vi "weather_update.vi"(2 "error in":errorcluster, 3 "Weather Configuration":string="{\n  \"set_profile\": \"CloudySunset\",\n  \"profiles\": [\n    {\n      \"id\": \"Default\",\n      \"SunPolarAngle\": 44.586,\n      \"SunAzimuthAngle\": 174,\n      \"SunBrightness\": 50,\n      \"SunDirectionalLightIntensity\": 15.092,\n      \"SunDirectionalLightColor\": {\n        \"R\": 255.0,\n        \"G\": 239.0,\n        \"B\": 194.0,\n        \"A\": 1.0\n      },\n      \"SunIndirectLightIntensity\": 6,\n      \"CloudOpacity\": 16.296,\n      \"HorizontFalloff\": 3,\n      \"ZenithColor\": {\n        \"R\": 0.034046,\n        \"G\": 0.109247,\n        \"B\": 0.295,\n        \"A\": 1.0\n      },\n      \"HorizonColor\": {\n        \"R\": 0.659853, \"G\": 0.862215, \"B\": 1.0, \"A\": 1.0\n      },\n      \"CloudColor\": {\n        \"R\": 0.855778, \"G\": 0.919005, \"B\": 1.0, \"A\": 1.0\n      },\n      \"OverallSkyColor\": {\n        \"R\": 1.0, \"G\": 1.0, \"B\": 1.0, \"A\": 1.0\n      },\n      \"SkyLightIntensity\": 5.505,\n      \"SkyLightColor\": {\n        \"R\":0.149650, \"G\":0.161819, \"B\":0.205000, \"A\":0.000000\n      },\n      \"bPrecipitation\": false,\n      \"PrecipitationType\": \"Rain\",\n      \"PrecipitationAmount\": 0,\n      \"PrecipitationAccumulation\": 0,\n      \"bWind\": false,\n      \"WindIntensity\": 20,\n      \"WindAngle\": 0,\n      \"bOverrideCameraPostProcessParameters\": true,\n      \"CameraPostProcessParameters\": {\n        \"AutoExposureMethod\": \"Histogram\",\n        \"AutoExposureMinBrightness\": 0.27,\n        \"AutoExposureMaxBrightness\": 5,\n        \"AutoExposureBias\": -3.5\n      }\n    },\n    {\n      \"id\": \"ClearNoon\",\n      \"SunPolarAngle\": 44.586,\n      \"SunAzimuthAngle\": 174,\n      \"SunBrightness\": 50,\n      \"SunDirectionalLightIntensity\": 34.286,\n      \"SunDirectionalLightColor\": {\"R\":255.000000, \"G\":239.000000, \"B\":194.000000, \"A\":1.0},\n      \"SunIndirectLightIntensity\": 6,\n      \"CloudOpacity\": 16.296,\n      \"HorizontFalloff\": 3,\n      \"ZenithColor\": {\"R\":0.034046, \"G\":0.109247, \"B\":0.295000, \"A\":1.0},\n      \"HorizonColor\": {\"R\":0.659853, \"G\":0.862215, \"B\":1.0, \"A\":1.0},\n      \"CloudColor\": {\"R\":0.855778, \"G\":0.919005, \"B\":1.0, \"A\":1.0},\n      \"OverallSkyColor\": {\"R\":1.0, \"G\":1.0, \"B\":1.0, \"A\":1.0},\n      \"SkyLightIntensity\": 10,\n      \"SkyLightColor\": {\"R\":0.195000, \"G\":0.193979, \"B\":0.152151, \"A\":0.000000},\n      \"bPrecipitation\": false,\n      \"PrecipitationType\": \"Rain\",\n      \"PrecipitationAmount\": 0,\n      \"PrecipitationAccumulation\": 0,\n      \"bWind\": false,\n      \"WindIntensity\": 20,\n      \"WindAngle\": 0,\n      \"bOverrideCameraPostProcessParameters\": true,\n      \"CameraPostProcessParameters\":{\n        \"AutoExposureMethod\": \"Histogram\",\n        \"AutoExposureMinBrightness\": 0.27,\n        \"AutoExposureMaxBrightness\": 5,\n        \"AutoExposureBias\": -3.5\n      }\n    },\n    {\n      \"id\": \"CloudyNoon\",\n      \"SunPolarAngle\": 44.586,\n      \"SunAzimuthAngle\": 174,\n      \"SunBrightness\": 0,\n      \"SunDirectionalLightIntensity\": 1.835,\n      \"SunDirectionalLightColor\": {\"R\":1.0, \"G\":0.862295, \"B\":0.475000, \"A\":1.0},\n      \"SunIndirectLightIntensity\": 6,\n      \"CloudOpacity\": 18.431,\n      \"HorizontFalloff\": 3,\n      \"ZenithColor\": {\"R\":1.0, \"G\":1.0, \"B\":1.0, \"A\":1.0},\n      \"HorizonColor\": {\"R\":0.169000, \"G\":0.187443, \"B\":0.200000, \"A\":1.0},\n      \"CloudColor\": {\"R\":0.143627, \"G\":0.159235, \"B\":0.190000, \"A\":1.0},\n      \"OverallSkyColor\": {\"R\":1.0, \"G\":1.0, \"B\":1.0, \"A\":1.0},\n      \"SkyLightIntensity\": 16.514,\n      \"SkyLightColor\": {\"R\":0.100887, \"G\":0.106803, \"B\":0.145000, \"A\":0.000000},\n      \"bPrecipitation\": false,\n      \"PrecipitationType\": \"Rain\",\n      \"PrecipitationAmount\": 0,\n      \"PrecipitationAccumulation\": 0,\n      \"bWind\": false,\n      \"WindIntensity\": 20,\n      \"WindAngle\": 0,\n      \"bOverrideCameraPostProcessParameters\": true,\n      \"CameraPostProcessParameters\": {\n        \"AutoExposureMethod\": \"Histogram\",\n        \"AutoExposureMinBrightness\": 0.27,\n        \"AutoExposureMaxBrightness\": 5,\n        \"AutoExposureBias\": -3.5\n      }\n    },\n    {\n      \"id\": \"WetNoon\",\n      \"SunPolarAngle\": 44.586,\n      \"SunAzimuthAngle\": 174,\n      \"SunBrightness\": 3.67,\n      \"SunDirectionalLightIntensity\": 20.184,\n      \"SunDirectionalLightColor\": {\"R\":1.0, \"G\":0.862295, \"B\":0.475000, \"A\":1.0},\n      \"SunIndirectLightIntensity\": 6,\n      \"CloudOpacity\": 17.431,\n      \"HorizontFalloff\": 5.752,\n      \"ZenithColor\": {\"R\":0.000000, \"G\":0.085618, \"B\":0.715000, \"A\":1.0},\n      \"HorizonColor\": {\"R\":0.532350, \"G\":0.590445, \"B\":0.630000, \"A\":1.0},\n      \"CloudColor\": {\"R\":0.143627, \"G\":0.159235, \"B\":0.190000, \"A\":1.0},\n      \"OverallSkyColor\": {\"R\":0.660000, \"G\":0.630413, \"B\":0.518100, \"A\":1.0},\n      \"SkyLightIntensity\": 14.679,\n      \"SkyLightColor\": {\"R\":0.135000, \"G\":0.120150, \"B\":0.075600, \"A\":0.000000},\n      \"bPrecipitation\": true,\n      \"PrecipitationType\": \"Rain\",\n      \"PrecipitationAmount\": 0,\n      \"PrecipitationAccumulation\": 54.128,\n      \"bWind\": false,\n      \"WindIntensity\": 20,\n      \"WindAngle\": 0,\n      \"bOverrideCameraPostProcessParameters\": true,\n      \"CameraPostProcessParameters\": {\n        \"AutoExposureMethod\": \"Histogram\",\n        \"AutoExposureMinBrightness\": 0.27,\n        \"AutoExposureMaxBrightness\": 5,\n        \"AutoExposureBias\": -3.5\n      }\n    },\n    {\n      \"id\": \"WetCloudyNoon\",\n      \"SunPolarAngle\": 44.586,\n      \"SunAzimuthAngle\": 174,\n      \"SunBrightness\": 0,\n      \"SunDirectionalLightIntensity\": 1.835,\n      \"SunDirectionalLightColor\": {\"R\":1.0, \"G\":0.862295, \"B\":0.475000, \"A\":1.0},\n      \"SunIndirectLightIntensity\": 6,\n      \"CloudOpacity\": 18.431,\n      \"HorizontFalloff\": 3,\n      \"ZenithColor\": {\"R\":1.0, \"G\":1.0, \"B\":1.0, \"A\":1.0},\n      \"HorizonColor\": {\"R\":0.000000, \"G\":0.000000, \"B\":0.000000, \"A\":1.0},\n      \"CloudColor\": {\"R\":0.230559, \"G\":0.255614, \"B\":0.305000, \"A\":1.0},\n      \"OverallSkyColor\": {\"R\":0.660000, \"G\":0.630413, \"B\":0.518100, \"A\":1.0},\n      \"SkyLightIntensity\": 25.688,\n      \"SkyLightColor\": {\"R\":0.135000, \"G\":0.120150, \"B\":0.075600, \"A\":0.000000},\n      \"bPrecipitation\": true,\n      \"PrecipitationType\": \"Rain\",\n      \"PrecipitationAmount\": 0,\n      \"PrecipitationAccumulation\": 47.706,\n      \"bWind\": false,\n      \"WindIntensity\": 20,\n      \"WindAngle\": 0,\n      \"bOverrideCameraPostProcessParameters\": true,\n      \"CameraPostProcessParameters\": {\n        \"AutoExposureMethod\": \"Histogram\",\n        \"AutoExposureMinBrightness\": 0.27,\n        \"AutoExposureMaxBrightness\": 5,\n        \"AutoExposureBias\": -3.5\n      }\n    },\n    {\n      \"id\": \"MidRainyNoon\",\n      \"SunPolarAngle\": 44.586,\n      \"SunAzimuthAngle\": 174,\n      \"SunBrightness\": 0,\n      \"SunDirectionalLightIntensity\": 1.33,\n      \"SunDirectionalLightColor\": {\"R\":255.000000, \"G\":239.000000, \"B\":194.000000, \"A\":1.0},\n      \"SunIndirectLightIntensity\": 6,\n      \"CloudOpacity\": 18.431,\n      \"HorizontFalloff\": 3,\n      \"ZenithColor\": {\"R\":0.370000, \"G\":0.370000, \"B\":0.370000, \"A\":1.0},\n      \"HorizonColor\": {\"R\":0.169000, \"G\":0.187443, \"B\":0.200000, \"A\":1.0},\n      \"CloudColor\": {\"R\":0.042789, \"G\":0.045950, \"B\":0.050000, \"A\":1.0},\n      \"OverallSkyColor\": {\"R\":1.0, \"G\":1.0, \"B\":1.0, \"A\":1.0},\n      \"SkyLightIntensity\": 21.147,\n      \"SkyLightColor\": {\"R\":0.119882, \"G\":0.121557, \"B\":0.170000, \"A\":0.000000},\n      \"bPrecipitation\": true,\n      \"PrecipitationType\": \"Rain\",\n      \"PrecipitationAmount\": 40,\n      \"PrecipitationAccumulation\": 50,\n      \"bWind\": false,\n      \"WindIntensity\": 40,\n      \"WindAngle\": 0,\n      \"bOverrideCameraPostProcessParameters\": true,\n      \"CameraPostProcessParameters\": {\n        \"AutoExposureMethod\": \"Histogram\",\n        \"AutoExposureMinBrightness\": 0.27,\n        \"AutoExposureMaxBrightness\": 5,\n        \"AutoExposureBias\": -3.5\n      }\n    },\n    {\n      \"id\": \"HardRainNoon\",\n      \"SunPolarAngle\": 44.586,\n      \"SunAzimuthAngle\": 174,\n      \"SunBrightness\": 0,\n      \"SunDirectionalLightIntensity\": 1.33,\n      \"SunDirectionalLightColor\": {\"R\":255.000000, \"G\":239.000000, \"B\":194.000000, \"A\":1.0},\n      \"SunIndirectLightIntensity\": 6,\n      \"CloudOpacity\": 18.431,\n      \"HorizontFalloff\": 3,\n      \"ZenithColor\": {\"R\":0.580000, \"G\":0.580000, \"B\":0.580000, \"A\":1.0},\n      \"HorizonColor\": {\"R\":0.169000, \"G\":0.187443, \"B\":0.200000, \"A\":1.0},\n      \"CloudColor\": {\"R\":0.089857, \"G\":0.096495, \"B\":0.105000, \"A\":1.0},\n      \"OverallSkyColor\": {\"R\":1.0, \"G\":1.0, \"B\":1.0, \"A\":1.0},\n      \"SkyLightIntensity\": 37.66,\n      \"SkyLightColor\": {\"R\":0.126934, \"G\":0.128707, \"B\":0.180000, \"A\":0.000000},\n      \"bPrecipitation\": true,\n      \"PrecipitationType\": \"Rain\",\n      \"PrecipitationAmount\": 80,\n      \"PrecipitationAccumulation\": 87.248,\n      \"bWind\": false,\n      \"WindIntensity\": 40,\n      \"WindAngle\": 0,\n      \"bOverrideCameraPostProcessParameters\": true,\n      \"CameraPostProcessParameters\": {\n        \"AutoExposureMethod\": \"Histogram\",\n        \"AutoExposureMinBrightness\": 0.27,\n        \"AutoExposureMaxBrightness\": 5,\n        \"AutoExposureBias\": -3.5\n      }\n    },\n    {\n      \"id\":\"SoftRainNoon\",\n      \"SunPolarAngle\": 44.586,\n      \"SunAzimuthAngle\": 174,\n      \"SunBrightness\": 0,\n      \"SunDirectionalLightIntensity\": 1.33,\n      \"SunDirectionalLightColor\": {\"R\":255.000000, \"G\":239.000000, \"B\":194.000000, \"A\":1.0},\n      \"SunIndirectLightIntensity\": 6,\n      \"CloudOpacity\": 18.431,\n      \"HorizontFalloff\": 3,\n      \"ZenithColor\": {\"R\":1.0, \"G\":1.0, \"B\":1.0, \"A\":1.0},\n      \"HorizonColor\": {\"R\":0.169000, \"G\":0.187443, \"B\":0.200000, \"A\":1.0},\n      \"CloudColor\": {\"R\":0.440725, \"G\":0.473285, \"B\":0.515000, \"A\":1.0},\n      \"OverallSkyColor\": {\"R\":1.0, \"G\":1.0, \"B\":1.0, \"A\":1.0},\n      \"SkyLightIntensity\": 3,\n      \"SkyLightColor\": {\"R\":0.525365, \"G\":0.532706, \"B\":0.745000, \"A\":0.000000},\n      \"bPrecipitation\": true,\n      \"PrecipitationType\": \"Rain\",\n      \"PrecipitationAmount\": 10.55,\n      \"PrecipitationAccumulation\": 61.927,\n      \"bWind\": false,\n      \"WindIntensity\": 20,\n      \"WindAngle\": 0,\n      \"bOverrideCameraPostProcessParameters\": true,\n      \"CameraPostProcessParameters\": {\n        \"AutoExposureMethod\": \"Histogram\",\n        \"AutoExposureMinBrightness\": 0.27,\n        \"AutoExposureMaxBrightness\": 5,\n        \"AutoExposureBias\": -3.5\n      }\n    },\n    {\n      \"id\": \"ClearSunset\",\n      \"SunPolarAngle\": 86,\n      \"SunAzimuthAngle\": 174,\n      \"SunBrightness\": 1.835,\n      \"SunDirectionalLightIntensity\": 50,\n      \"SunDirectionalLightColor\": {\"R\":0.810000, \"G\":0.347470, \"B\":0.170100, \"A\":1.0},\n      \"SunIndirectLightIntensity\": 73.394,\n      \"CloudOpacity\": 27.63,\n      \"HorizontFalloff\": 0.917,\n      \"ZenithColor\": {\"R\":0.046375, \"G\":0.044100, \"B\":0.105000, \"A\":1.0},\n      \"HorizonColor\": {\"R\":0.745000, \"G\":0.219006, \"B\":0.046649, \"A\":1.0},\n      \"CloudColor\": {\"R\":1.0, \"G\":0.561587, \"B\":0.189305, \"A\":1.0},\n      \"OverallSkyColor\": {\"R\":1.0, \"G\":1.0, \"B\":1.0, \"A\":1.0},\n      \"SkyLightIntensity\": 14,\n      \"SkyLightColor\": {\"R\":0.076220, \"G\":0.074724, \"B\":0.109375, \"A\":0.000000},\n      \"bPrecipitation\": false,\n      \"PrecipitationType\": \"Rain\",\n      \"PrecipitationAmount\": 0,\n      \"PrecipitationAccumulation\": 0,\n      \"bWind\": false,\n      \"WindIntensity\": 20,\n      \"WindAngle\": 0,\n      \"bOverrideCameraPostProcessParameters\": true,\n      \"CameraPostProcessParameters\": {\n        \"AutoExposureMethod\": \"Histogram\",\n        \"AutoExposureMinBrightness\": 0.27,\n        \"AutoExposureMaxBrightness\": 5,\n        \"AutoExposureBias\": -3.5\n      }\n    },\n    {\n      \"id\": \"CloudySunset\",\n      \"SunPolarAngle\": 86,\n      \"SunAzimuthAngle\": 174,\n      \"SunBrightness\": 67.89,\n      \"SunDirectionalLightIntensity\": 6.422,\n      \"SunDirectionalLightColor\": {\"R\":0.810000, \"G\":0.347162, \"B\":0.083003, \"A\":1.0},\n      \"SunIndirectLightIntensity\": 6,\n      \"CloudOpacity\": 28.869,\n      \"HorizontFalloff\": 1.165,\n      \"ZenithColor\": {\"R\":0.046375, \"G\":0.044100, \"B\":0.105000, \"A\":1.0},\n      \"HorizonColor\": {\"R\":1.0, \"G\":0.007579, \"B\":0.000000, \"A\":1.0},\n      \"CloudColor\": {\"R\":1.0, \"G\":0.518982, \"B\":0.175000, \"A\":1.0},\n      \"OverallSkyColor\": {\"R\":0.410000, \"G\":0.410000, \"B\":0.410000, \"A\":1.0},\n      \"SkyLightIntensity\": 36.239,\n      \"SkyLightColor\": {\"R\":0.193050, \"G\":0.195113, \"B\":0.270000, \"A\":0.000000},\n      \"bPrecipitation\": false,\n      \"PrecipitationType\": \"Rain\",\n      \"PrecipitationAmount\": 0,\n      \"PrecipitationAccumulation\": 0,\n      \"bWind\": false,\n      \"WindIntensity\": 20,\n      \"WindAngle\": 0,\n      \"bOverrideCameraPostProcessParameters\": true,\n      \"CameraPostProcessParameters\": {\n        \"AutoExposureMethod\": \"Histogram\",\n        \"AutoExposureMinBrightness\": 0.27,\n        \"AutoExposureMaxBrightness\": 5,\n        \"AutoExposureBias\": -3.5\n      }\n    },\n    {\n      \"id\": \"WetSunset\",\n      \"SunPolarAngle\": 86,\n      \"SunAzimuthAngle\": 174,\n      \"SunBrightness\": 0,\n      \"SunDirectionalLightIntensity\": 25.688,\n      \"SunDirectionalLightColor\": {\"R\":0.810000, \"G\":0.347162, \"B\":0.083003, \"A\":1.0},\n      \"SunIndirectLightIntensity\": 6,\n      \"CloudOpacity\": 17.596,\n      \"HorizontFalloff\": 1.165,\n      \"ZenithColor\": {\"R\":0.046375, \"G\":0.044100, \"B\":0.105000, \"A\":1.0},\n      \"HorizonColor\": {\"R\":0.695000, \"G\":0.379445, \"B\":0.150922, \"A\":1.0},\n      \"CloudColor\": {\"R\":1.0, \"G\":0.561587, \"B\":0.189305, \"A\":1.0},\n      \"OverallSkyColor\": {\"R\":1.0, \"G\":1.0, \"B\":1.0, \"A\":1.0},\n      \"SkyLightIntensity\": 66.972,\n      \"SkyLightColor\": {\"R\":0.113887, \"G\":0.110000, \"B\":0.200000, \"A\":0.000000},\n      \"bPrecipitation\": true,\n      \"PrecipitationType\": \"Rain\",\n      \"PrecipitationAmount\": 0,\n      \"PrecipitationAccumulation\": 65.046,\n      \"bWind\": false,\n      \"WindIntensity\": 20,\n      \"WindAngle\": 0,\n      \"bOverrideCameraPostProcessParameters\": true,\n      \"CameraPostProcessParameters\": {\n        \"AutoExposureMethod\": \"Histogram\",\n        \"AutoExposureMinBrightness\": 0.27,\n        \"AutoExposureMaxBrightness\": 5,\n        \"AutoExposureBias\": -3.5\n      }\n    },\n    {\n      \"id\": \"WetCloudySunset\",\n      \"SunPolarAngle\": 86,\n      \"SunAzimuthAngle\": 174,\n      \"SunBrightness\": 67.89,\n      \"SunDirectionalLightIntensity\": 25.688,\n      \"SunDirectionalLightColor\": {\"R\":0.810000, \"G\":0.347162, \"B\":0.083003, \"A\":1.0},\n      \"SunIndirectLightIntensity\": 6,\n      \"CloudOpacity\": 15,\n      \"HorizontFalloff\": 1.165,\n      \"ZenithColor\": {\"R\":0.046375, \"G\":0.044100, \"B\":0.105000, \"A\":1.0},\n      \"HorizonColor\": {\"R\":0.695000, \"G\":0.379445, \"B\":0.150922, \"A\":1.0},\n      \"CloudColor\": {\"R\":1.0, \"G\":0.561587, \"B\":0.189305, \"A\":1.0},\n      \"OverallSkyColor\": {\"R\":1.0, \"G\":1.0, \"B\":1.0, \"A\":1.0},\n      \"SkyLightIntensity\": 50,\n      \"SkyLightColor\": {\"R\":0.083625, \"G\":0.081983, \"B\":0.120000, \"A\":0.000000},\n      \"bPrecipitation\": false,\n      \"PrecipitationType\": \"Rain\",\n      \"PrecipitationAmount\": 0,\n      \"PrecipitationAccumulation\": 0,\n      \"bWind\": false,\n      \"WindIntensity\": 20,\n      \"WindAngle\": 0,\n      \"bOverrideCameraPostProcessParameters\": true,\n      \"CameraPostProcessParameters\": {\n        \"AutoExposureMethod\": \"Histogram\",\n        \"AutoExposureMinBrightness\": 0.27,\n        \"AutoExposureMaxBrightness\": 5,\n        \"AutoExposureBias\": -3.5\n      }\n    },\n    {\n      \"id\": \"MidRainSunset\",\n      \"SunPolarAngle\": 86,\n      \"SunAzimuthAngle\": 174,\n      \"SunBrightness\": 12.381,\n      \"SunDirectionalLightIntensity\": 5.714,\n      \"SunDirectionalLightColor\": {\"R\":0.810000, \"G\":0.347162, \"B\":0.083003, \"A\":1.0},\n      \"SunIndirectLightIntensity\": 6,\n      \"CloudOpacity\": 17.143,\n      \"HorizontFalloff\": 1.835,\n      \"ZenithColor\": {\"R\":0.317708, \"G\":0.208096, \"B\":0.260868, \"A\":1.0},\n      \"HorizonColor\": {\"R\":1.0, \"G\":0.590000, \"B\":0.000000, \"A\":1.0},\n      \"CloudColor\": {\"R\":0.555000, \"G\":0.290880, \"B\":0.066600, \"A\":1.0},\n      \"OverallSkyColor\": {\"R\":1.0, \"G\":1.0, \"B\":1.0, \"A\":1.0},\n      \"SkyLightIntensity\": 6.667,\n      \"SkyLightColor\": {\"R\":0.214844, \"G\":0.273773, \"B\":0.750000, \"A\":0.000000},\n      \"bPrecipitation\": true,\n      \"PrecipitationType\": \"Rain\",\n      \"PrecipitationAmount\": 37.156,\n      \"PrecipitationAccumulation\": 88.073,\n      \"bWind\": false,\n      \"WindIntensity\": 20,\n      \"WindAngle\": 0,\n      \"bOverrideCameraPostProcessParameters\": true,\n      \"CameraPostProcessParameters\": {\n        \"AutoExposureMethod\": \"Histogram\",\n        \"AutoExposureMinBrightness\": 0.27,\n        \"AutoExposureMaxBrightness\": 5,\n        \"AutoExposureBias\": -3.5\n      }\n    },\n    {\n      \"id\": \"HardRainSunset\",\n      \"SunPolarAngle\": 86,\n      \"SunAzimuthAngle\": 174,\n      \"SunBrightness\": 0.952,\n      \"SunDirectionalLightIntensity\": 3.063,\n      \"SunDirectionalLightColor\": {\"R\":0.810000, \"G\":0.347162, \"B\":0.083003, \"A\":1.0},\n      \"SunIndirectLightIntensity\": 6,\n      \"CloudOpacity\": 17.37,\n      \"HorizontFalloff\": 1.835,\n      \"ZenithColor\": {\"R\":0.307292, \"G\":0.161669, \"B\":0.123237, \"A\":1.0},\n      \"HorizonColor\": {\"R\":0.453125, \"G\":0.297809, \"B\":0.228923, \"A\":1.0},\n      \"CloudColor\": {\"R\":0.416667, \"G\":0.288257, \"B\":0.189558, \"A\":1.0},\n      \"OverallSkyColor\": {\"R\":1.0, \"G\":0.736403, \"B\":0.487039, \"A\":1.0},\n      \"SkyLightIntensity\": 5.81,\n      \"SkyLightColor\": {\"R\":0.500000, \"G\":0.383356, \"B\":0.250000, \"A\":0.000000},\n      \"bPrecipitation\": true,\n      \"PrecipitationType\": \"Rain\",\n      \"PrecipitationAmount\": 84.862,\n      \"PrecipitationAccumulation\": 100,\n      \"bWind\": false,\n      \"WindIntensity\": 20,\n      \"WindAngle\": 0,\n      \"bOverrideCameraPostProcessParameters\": true,\n      \"CameraPostProcessParameters\": {\n        \"AutoExposureMethod\": \"Histogram\",\n        \"AutoExposureMinBrightness\": 0.27,\n        \"AutoExposureMaxBrightness\": 5,\n        \"AutoExposureBias\": -3.5\n      }\n    },\n    {\n      \"id\": \"SoftRainSunset\",\n      \"SunPolarAngle\": 86,\n      \"SunAzimuthAngle\": 174,\n      \"SunBrightness\": 13.761,\n      \"SunDirectionalLightIntensity\": 12.587,\n      \"SunDirectionalLightColor\": {\"R\":0.810000, \"G\":0.347162, \"B\":0.083003, \"A\":1.0},\n      \"SunIndirectLightIntensity\": 6,\n      \"CloudOpacity\": 34.513,\n      \"HorizontFalloff\": 1.835,\n      \"ZenithColor\": {\"R\":0.360000, \"G\":0.125625, \"B\":0.142175, \"A\":1.0},\n      \"HorizonColor\": {\"R\":1.0, \"G\":0.590000, \"B\":0.000000, \"A\":1.0},\n      \"CloudColor\": {\"R\":0.296875, \"G\":0.169776, \"B\":0.061849, \"A\":1.0},\n      \"OverallSkyColor\": {\"R\":1.0, \"G\":1.0, \"B\":1.0, \"A\":1.0},\n      \"SkyLightIntensity\": 7.339,\n      \"SkyLightColor\": {\"R\":0.458070, \"G\":0.394209, \"B\":0.750000, \"A\":0.000000},\n      \"bPrecipitation\": true,\n      \"PrecipitationType\": \"Rain\",\n      \"PrecipitationAmount\": 8.716,\n      \"PrecipitationAccumulation\": 53.211,\n      \"bWind\": false,\n      \"WindIntensity\": 20,\n      \"WindAngle\": 0,\n      \"bOverrideCameraPostProcessParameters\": true,\n      \"CameraPostProcessParameters\": {\n        \"AutoExposureMethod\": \"Histogram\",\n        \"AutoExposureMinBrightness\": 0.27,\n        \"AutoExposureMaxBrightness\": 5,\n        \"AutoExposureBias\": -3.5\n      }\n    }\n  ]\n}\n", 4 "simx in":T1={"Config"={"Trajectory"={"Number of frames"=0, "Frame number"=0, "Trajectory"=""}, "Weather"={"id"=""}}, "Connections"={"Simulator Connection"=refnum, "server_ip"="127.0.0.1", "Port"=0, "Sensor connections"=[]}, "Map"={"lanes"={"x"=[], "y"=[], "z"=[]}, "StartPosition"={"start_points"={"locations"=[], "rotations"=[], "type"=[]}, "StartRotation"=[], "StartLocation"=[]}, "Draw Map Size"={"Width"=0, "Height"=0}, "DrawArea"={"min_Y"=0.0, "min_X"=0.0, "Scale X"=0.0, "Scale Y"=0.0}, "Map"=bytes[0], "Map Geojson"=""}}) -> (0 "error out":errorcluster, 1 "simx out":T1={"Config"={"Trajectory"={"Number of frames"=0, "Frame number"=0, "Trajectory"=""}, "Weather"={"id"=""}}, "Connections"={"Simulator Connection"=refnum, "server_ip"="127.0.0.1", "Port"=0, "Sensor connections"=[]}, "Map"={"lanes"={"x"=[], "y"=[], "z"=[]}, "StartPosition"={"start_points"={"locations"=[], "rotations"=[], "type"=[]}, "StartRotation"=[], "StartLocation"=[]}, "Draw Map Size"={"Width"=0, "Height"=0}, "DrawArea"={"min_Y"=0.0, "min_X"=0.0, "Scale X"=0.0, "Scale Y"=0.0}, "Map"=bytes[0], "Map Geojson"=""}})   [LabVIEW 2019, in "Lib_Simx.lvlib"]
doc: "Sends weather configuration to the simulator."
uses:
  Lib_Simx.lvlib
  controls/simx_connection.ctl
  controls/config.ctl
  controls/trajectory.ctl
  controls/weather.ctl
  controls/connections.ctl
  controls/start_points.ctl
  <vilib>/Utility/miscctls.llb/LVBoundsTypeDef.ctl
panel:
  out "JSON string":string
  out "weather updated":bool
  out "config response":string
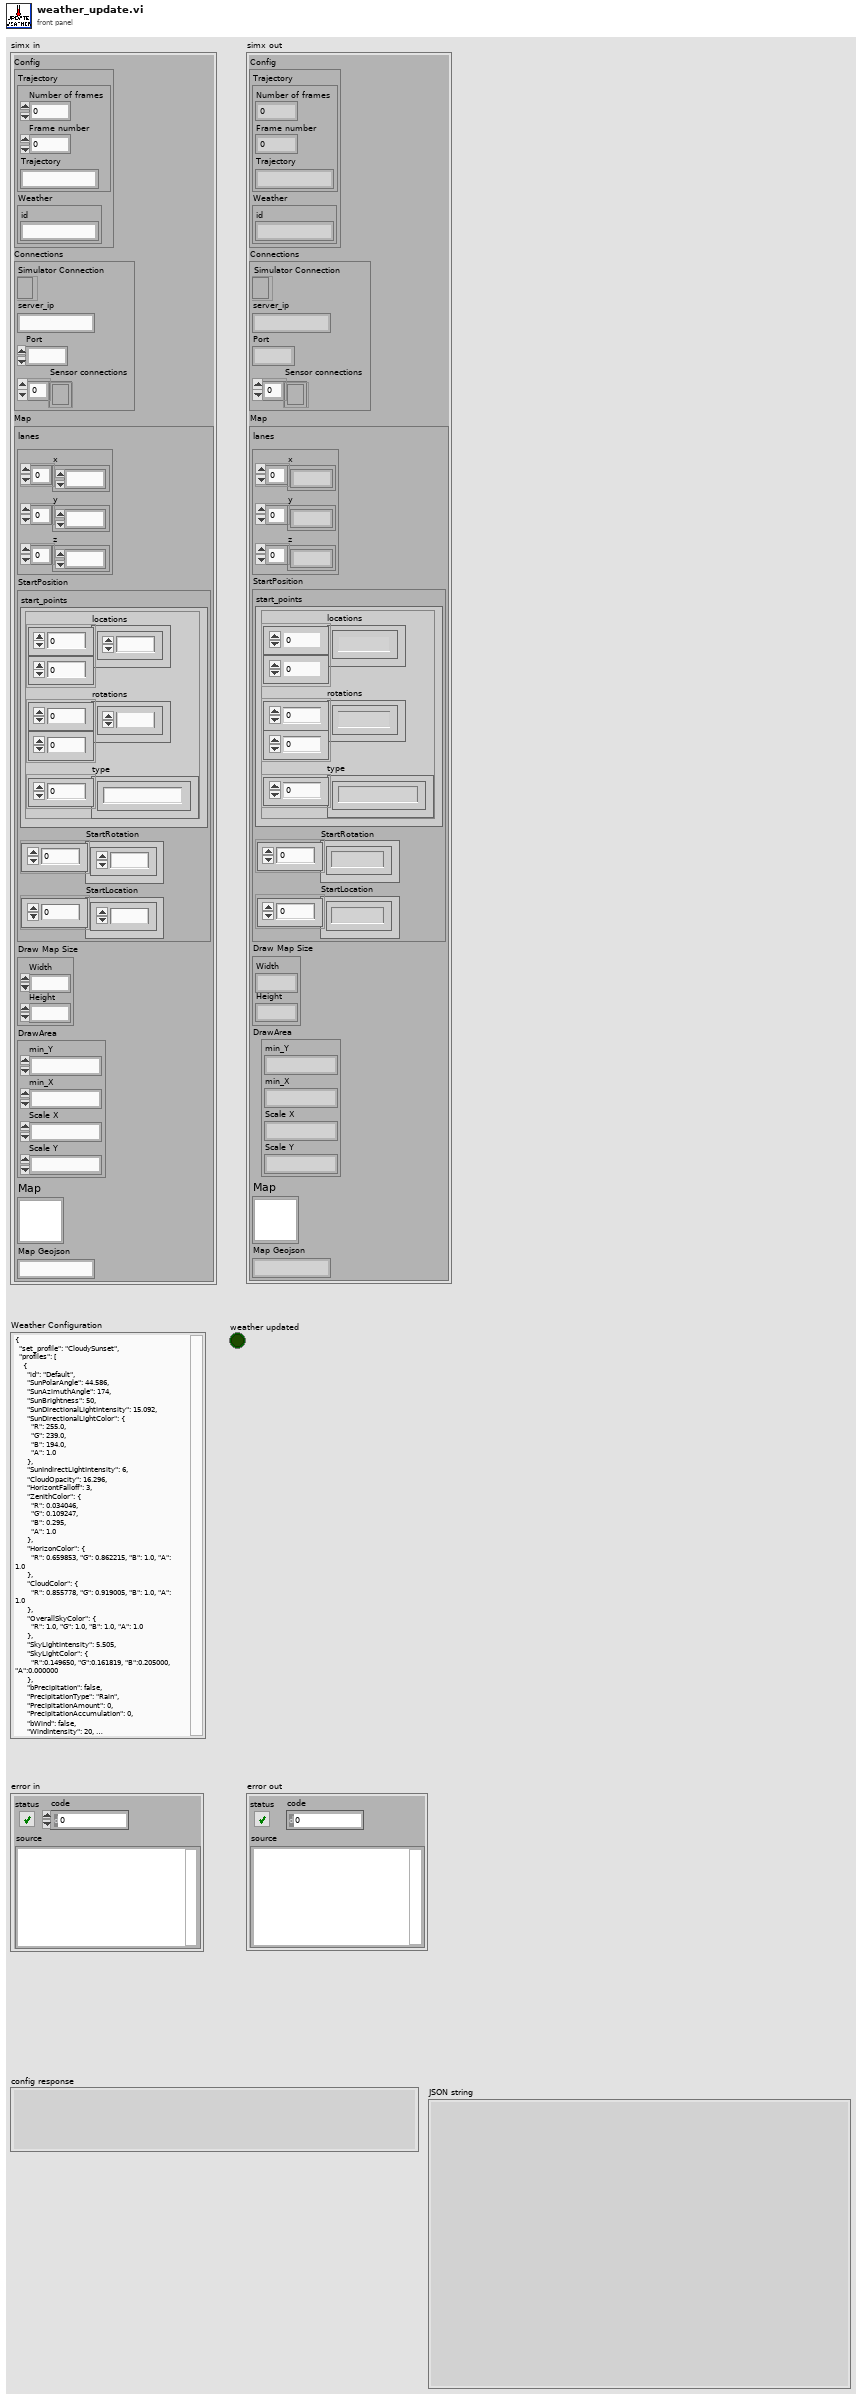
[diagram p1: front panel]
types:
  T1 = typedef "Lib_Simx.lvlib/simx_connection.ctl" = cluster{"Config":T2, "Connections":T5, "Map":cluster{"lanes":cluster{"x":dbl[], "y":dbl[], "z":dbl[]}, "StartPosition":cluster{"start_points":T6, "StartRotation":dbl[], "StartLocation":dbl[]}, "Draw Map Size":T7, "DrawArea":cluster{"min_Y":dbl, "min_X":dbl, "Scale X":dbl, "Scale Y":dbl}, "Map":picture, "Map Geojson":string}}
  T2 = typedef "Lib_Simx.lvlib/config.ctl" = cluster{"Trajectory":T3, "Weather":T4}
  T3 = typedef "Lib_Simx.lvlib/trajectory.ctl" = cluster{"Number of frames":i32, "Frame number":i32, "Trajectory":string}
  T4 = typedef "Lib_Simx.lvlib/weather.ctl" = cluster{"id":string}
  T5 = typedef "Lib_Simx.lvlib/connections.ctl" = cluster{"Simulator Connection":refnum<k5>, "server_ip":string, "Port":i32, "Sensor connections":refnum<k5>[]}
  T6 = typedef "Lib_Simx.lvlib/start_points.ctl" = cluster{"locations":dbl[][], "rotations":dbl[][], "type":string[]}
  T7 = typedef "LVBoundsTypeDef.ctl" = cluster{"Width":u32, "Height":u32}
  T8 = cluster{"set_description":string, "descriptions":cluster{"id":string, "CloudColor":cluster{"A":sgl, "B":sgl, "G":sgl, "R":sgl}, "CloudOpacity":sgl, "Day":sgl, "FogCutoffDistance":sgl, "FogDensity":sgl, "FogHeightFalloff":sgl, "FogInscatteringColor":cluster{"A":sgl, "B":sgl, "G":sgl, "R":sgl}, "FogMaxOpacity":sgl, "FogStartDistance":sgl, "HorizonColor":cluster{"A":sgl, "B":sgl, "G":sgl, "R":sgl}, "HorizonFalloff":sgl, "Hours":sgl, "IsDaylightSavingTime":bool, "Latitude":sgl, "Longitude":sgl, "Minutes":sgl, "Month":sgl, "NorthOffset":sgl, "OverallSkyColor":cluster{"A":sgl, "B":sgl, "G":sgl, "R":sgl}, "OverideTimeBasedSunAngle":bool, "PrecipitationAccumulation":sgl, "PrecipitationAmount":sgl, "PrecipitationType":string, "SecondFogDensity":sgl, "SecondFogHeightFalloff":sgl, "SecondFogHeightOffset":sgl, "Seconds":sgl, "SkyLightColor":cluster{"A":sgl, "B":sgl, "G":sgl, "R":sgl}, "SkyLightIntensity":sgl, "StarBrightness":sgl, "SunAzimuthAngle":sgl, "SunBrightness":sgl, "SunDirectionalLightColor":cluster{"A":sgl, "B":sgl, "G":sgl, "R":sgl}, "SunDirectionalLightIntensity":sgl, "SunPolarAngle":sgl, "TimeZone":sgl, "WindAngle":sgl, "WindIntensity":sgl, "Year":sgl, "ZenithColor":cluster{"A":sgl, "B":sgl, "G":sgl, "R":sgl}, "bPrecipitation":bool, "bWind":bool}[]}
  T9 = cluster{"type":string, "success":bool, "reference":i32}
  T10 = cluster{"id":string, "CloudColor":cluster{"A":sgl, "B":sgl, "G":sgl, "R":sgl}, "CloudOpacity":sgl, "Day":sgl, "FogCutoffDistance":sgl, "FogDensity":sgl, "FogHeightFalloff":sgl, "FogInscatteringColor":cluster{"A":sgl, "B":sgl, "G":sgl, "R":sgl}, "FogMaxOpacity":sgl, "FogStartDistance":sgl, "HorizonColor":cluster{"A":sgl, "B":sgl, "G":sgl, "R":sgl}, "HorizonFalloff":sgl, "Hours":sgl, "IsDaylightSavingTime":bool, "Latitude":sgl, "Longitude":sgl, "Minutes":sgl, "Month":sgl, "NorthOffset":sgl, "OverallSkyColor":cluster{"A":sgl, "B":sgl, "G":sgl, "R":sgl}, "OverideTimeBasedSunAngle":bool, "PrecipitationAccumulation":sgl, "PrecipitationAmount":sgl, "PrecipitationType":string, "SecondFogDensity":sgl, "SecondFogHeightFalloff":sgl, "SecondFogHeightOffset":sgl, "Seconds":sgl, "SkyLightColor":cluster{"A":sgl, "B":sgl, "G":sgl, "R":sgl}, "SkyLightIntensity":sgl, "StarBrightness":sgl, "SunAzimuthAngle":sgl, "SunBrightness":sgl, "SunDirectionalLightColor":cluster{"A":sgl, "B":sgl, "G":sgl, "R":sgl}, "SunDirectionalLightIntensity":sgl, "SunPolarAngle":sgl, "TimeZone":sgl, "WindAngle":sgl, "WindIntensity":sgl, "Year":sgl, "ZenithColor":cluster{"A":sgl, "B":sgl, "G":sgl, "R":sgl}, "bPrecipitation":bool, "bWind":bool}[]
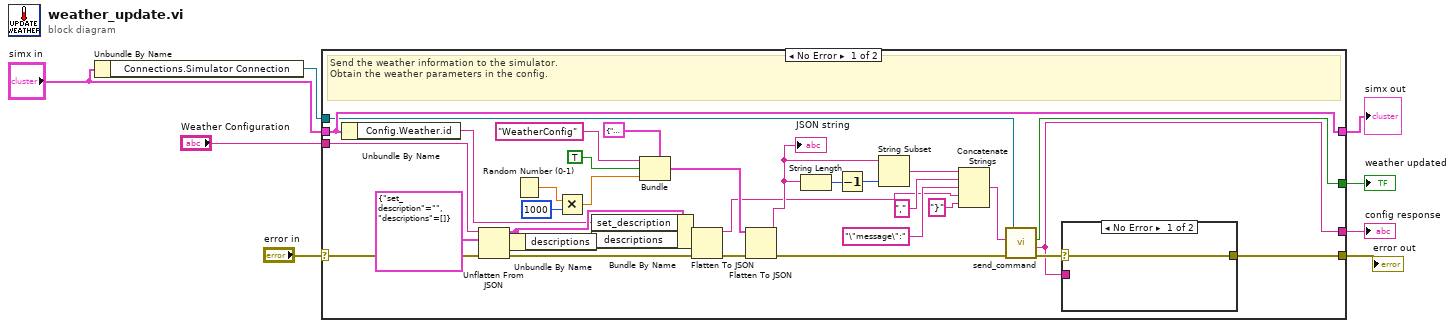
[diagram p0: block diagram]
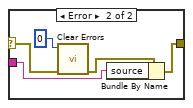
[diagram p2: hidden frame]
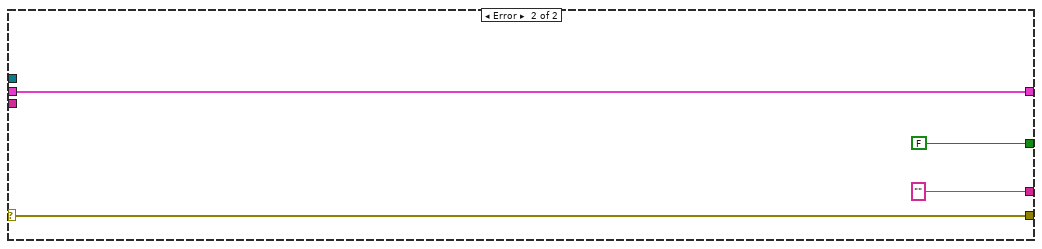
[diagram p3: hidden frame]
diagram:
  n1 = Unbundle By Name("simx in") -> ("Connections.Simulator Connection"=w2:refnum<k5>)
  n2 = case shown="No Error" "error in" {
    selector: "error in" -> [w13 w50]
    tunnel: [w29 "" ("response")] -> w8
    tunnel: [w30 w50] -> w7
    tunnel: [w32 FALSE ("success")] -> w5
    tunnel: "simx in" -> [w35 w47]
    tunnel: [w35 w47] -> w4
    tunnel: w2 -> [w34 _]
    tunnel: "Weather Configuration" -> [w19 _]
    frame No Error {
      # "Send the weather information to the simulator. \nObtain the weather parameters in the config."
      n3 = Unbundle By Name(w35) -> ("Config.Weather.id"=w16:string)
      n4 = Unflatten From JSON(JSON string=w19, type and defaults=T8 {"set_description"="", "descriptions"=[]}, error in (no error)=w13) -> (value=w18:T8, error out=w12:errorcluster)  [unwired: 4 in]
      n5 = Unbundle By Name(w18) -> ("descriptions"=w17:T10)
      n6 = Random Number (0-1)() -> (number: 0 to 1=w40:dbl)
      n7 = Multiply(x=w40, y=1000) -> (x*y=w37:dbl)
      n8 = Bundle By Name(cluster=w18, "set_description"=w16, "descriptions"=w17) -> (w15:T8)
      n9 = Bundle(cluster=T9 {"type"="", "success"=TRUE, "reference"=0}, "type"="WeatherConfig" ("Command_ID"), "success"=TRUE, "reference"=w37) -> (w28:T9)
      n10 = Flatten To JSON(anything=w15, error in (no error)=w12) -> (JSON string=w14:string, 11:w11:errorcluster)  [unwired: 1 in]
      n11 = Flatten To JSON(anything=w28, error in (no error)=w11) -> (JSON string=w25:string, 11:w33:errorcluster)  [unwired: 1 in]
      "JSON string" <- w25
      n12 = String Length(string=w25) -> (length=w26:i32)
      n13 = Decrement(x=w26) -> (x-1=w24:i32)
      n14 = String Subset(string=w25, length (rest)=w24) -> (substring=w27:string)  [unwired: 1 in]
      n15 = Concatenate Strings(w27, "," ("string"), "\"message\":" ("string"), w14, "}" ("string")) -> (w23:string)
      n16 = call "send_command.vi"("error in"=w33, "JSON Command"=w23, "TCP Network Connection in"=w34) -> ("error out"=w31:errorcluster, "Response"=w29:string, "Success"=w32:bool)  [unwired: 1 in, 1 out]
      n17 = case shown="No Error" w31 {
        selector: w31 -> [w41 w43]
        tunnel: [w41 w46] -> w30
        tunnel: w29 -> [_ w45]
        frame No Error {
        }
        frame Error {
          n18 = call <vilib>:"Clear Errors.vi"("error in (no error)"=w43, "specific error code to clear (0: all)"=0) -> ("error out"=w42:errorcluster)  [unwired: 4 in, 1 out]
          n19 = Bundle By Name(cluster=w42, "source"=w45) -> (w46:errorcluster)
        }
      }
    }
    frame Error {
    }
  }
  "config response" <- w8
  "error out" <- w7
  "weather updated" <- w5
  "simx out" <- w4
